vi "Read TransparentColor.vi"(8 "error in (no error)":errorcluster, 11 "RT_Sprite in":refnum<class "RT_Sprite.lvclass">) -> (0 "error out":errorcluster, 2 "TransparentColor":fxp<+,3,3>, 3 "RT_Sprite out":refnum<class "RT_Sprite.lvclass">)   [LabVIEW 2019, in "RT_Game.lvlib" / "RT_Sprite.lvclass"]
uses:
  RT_Sprite.lvclass
  RT_Sprite.lvclass/RT_Sprite.ctl
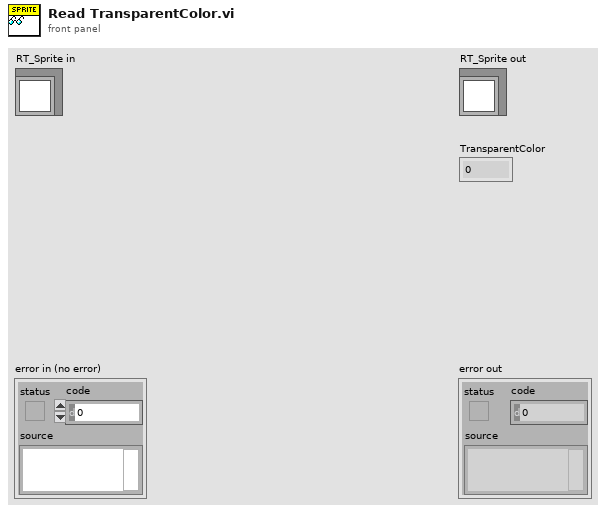
[diagram p1: front panel]
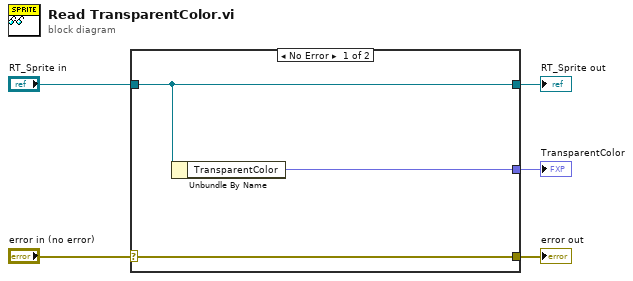
[diagram p0: block diagram]
diagram:
  n1 = case shown="No Error" "error in (no error)" {
    selector: "error in (no error)" -> [w8 w9]
    tunnel: [w8 w9] -> w4
    tunnel: [w7 w10] -> w2
    tunnel: "RT_Sprite in" -> [w7 w10]
    tunnel: [w6 _] -> w1
    frame No Error {
      n2 = Unbundle By Name(w7) -> ("TransparentColor"=w6:fxp<+,3,3>)
    }
    frame Error {
    }
  }
  "error out" <- w4
  "RT_Sprite out" <- w2
  "TransparentColor" <- w1
